vi "PH_Calorimeter_USB.get Data.vi"(0 "i ref in":refnum<vi>, 5 "error in (no error)":errorcluster) -> (14 "i ref out":refnum<vi>, 16 "raw data":dbl[][](array[numeric]), 17 "got Data":bool, 19 "error out":errorcluster)   [LabVIEW 2014, in "PH_Calorimeter_USB.lvlib"]
doc: "This VI interacts with the hardware. The data are taken and written to own attributes and the GUI."
uses:
  PH_Calorimeter_USB.lvlib
  <vilib>/DAQmx/create/channels.llb/DAQmx Create Channel (AI-Voltage-Basic).vi
  <vilib>/DAQmx/configure/timing.llb/DAQmx Timing (Sample Clock).vi
  <vilib>/DAQmx/read.llb/DAQmx Read (Analog 2D DBL NChan NSamp).vi
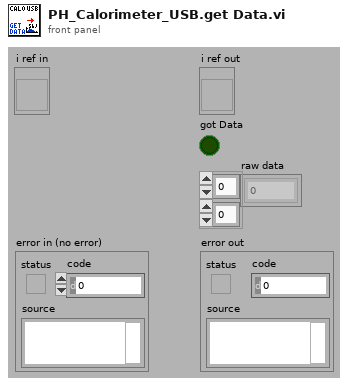
[diagram p1: front panel]
types:
  T1 = typedef "PH_Calorimeter_USB.lvlib/PH_Calorimeter_USB.i attribute.ctl" = cluster{"GUI Refs":cluster{"Delete":refnum<vi>, "Start":refnum<vi>, "Energy":refnum<vi>, "Calorimeter":refnum<vi>, "Trigger":refnum<vi>, "Calo Calibration":refnum<vi>, "Time Base":refnum<vi>, "Device":refnum<vi>, "Graph Raw Data":refnum<vi>, "Graph Result":refnum<vi>}, "DAQ Instance":string, "Data":dbl[][], "Controller Instance":string, "Energy [J]":dbl, "Calorimeter":T2, "Trigger":T3, "Time Base":T4, "Calo Calibration":T5, "Serial Number":string}
  T2 = typedef "PH_Calorimeter_USB.lvlib/PH_Calorimeter_USB.Calorimeter Settings.ctl" = cluster{"Channel":tag, "Min Value [V]":dbl, "Max Value  [V]":dbl}
  T3 = typedef "PH_Calorimeter_USB.lvlib/PH_Calorimeter_USB.Trigger Settings.ctl" = cluster{"Channel":tag, "Min Value [V]":dbl, "Max Value  [V]":dbl, "Level [V]":dbl, "Wait Time [s]":dbl, "Length [Samples]":i32}
  T4 = typedef "PH_Calorimeter_USB.lvlib/PH_Calorimeter_USB.Time Base Settings.ctl" = cluster{"Samples per Channel":i32, "Rate [Hz]":i32}
  T5 = typedef "PH_Calorimeter_USB.lvlib/PH_Calorimeter_USB.Calorimeter Calibration Settings.ctl" = cluster{"T 1/e [s]":dbl, "Sensitivity  [Vs/J]":dbl}
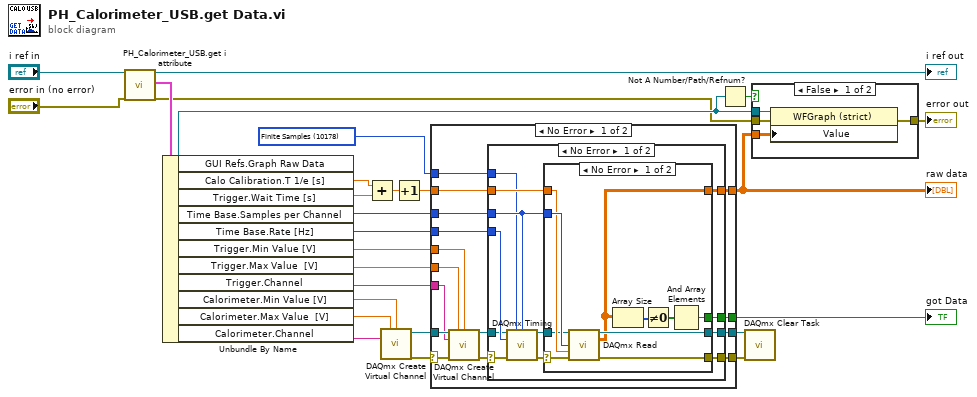
[diagram p0: block diagram]
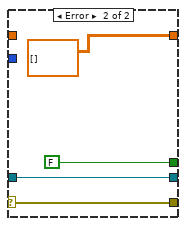
[diagram p2: hidden frame]
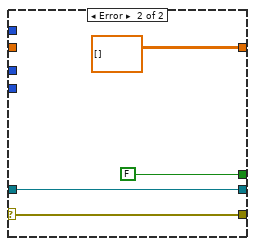
[diagram p3: hidden frame]
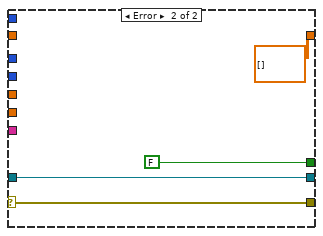
[diagram p4: hidden frame]
diagram:
  w3 = 10178 items=["Finite Samples"=10178, "Continuous Samples"=10123] ("sample mode")
  n1 = call "PH_Calorimeter_USB.get i attribute.vi"("i ref in"="i ref in", "error in (no error)"="error in (no error)") -> ("i ref out"=→"i ref out":refnum<vi>, "i attribute"=w16:T1, "error out"=w8:errorcluster)  [unwired: 15 in]
  n2 = Unbundle By Name(w16) -> ("GUI Refs.Graph Raw Data"=w27:refnum<vi>, "Calo Calibration.T 1/e [s]"=w25:dbl, "Trigger.Wait Time [s]"=w24:dbl, "Time Base.Samples per Channel"=w23:i32, "Time Base.Rate [Hz]"=w22:i32, "Trigger.Min Value [V]"=w21:dbl, "Trigger.Max Value  [V]"=w20:dbl, "Trigger.Channel"=w6:tag, "Calorimeter.Min Value [V]"=w19:dbl, "Calorimeter.Max Value  [V]"=w18:dbl, "Calorimeter.Channel"=w17:tag)
  n3 = Add(x=w25, y=w24) -> (x+y=w12:dbl)
  n4 = call-poly <vilib>:"DAQmx Create Virtual Channel.vi"("maximum value"=w18, "minimum value"=w19, "physical channels"=w17) -> ("task out"=w9:refnum<k21>, "error out"=w5:errorcluster)  [unwired: 11 in]
  n5 = Increment(x=w12) -> (x+1=w13:dbl)
  n6 = case shown="No Error" w5 {
    selector: w5 -> [w31 w76]
    tunnel: w23 -> [w42 _]
    tunnel: w22 -> [w41 _]
    tunnel: w21 -> [w40 _]
    tunnel: w20 -> [w39 _]
    tunnel: w13 -> [w38 _]
    tunnel: [w37 w75] -> w11
    tunnel: [w36 w76] -> w10
    tunnel: w9 -> [w35 w75]
    tunnel: [w34 dbl[][] [] ("data")] -> w7
    tunnel: w6 -> [w33 _]
    tunnel: [w29 FALSE] -> w4
    tunnel: w3 -> [w28 _]
    frame No Error {
      n7 = call-poly <vilib>:"DAQmx Create Virtual Channel.vi"("task in"=w35, "maximum value"=w39, "minimum value"=w40, "physical channels"=w33, "error in"=w31) -> ("task out"=w32:refnum<k21>, "error out"=w30:errorcluster)  [unwired: 9 in]
      n8 = case shown="No Error" w30 {
        selector: w30 -> [w46 w70]
        tunnel: w42 -> [w54 _]
        tunnel: w41 -> [w53 _]
        tunnel: w38 -> [w52 _]
        tunnel: [w51 w69] -> w37
        tunnel: [w50 w70] -> w36
        tunnel: [w49 dbl[][] [] ("data")] -> w34
        tunnel: w32 -> [w47 w69]
        tunnel: [w44 FALSE] -> w29
        tunnel: w28 -> [w43 _]
        frame No Error {
          n9 = call-poly <vilib>:"DAQmx Timing.vi"("task/channels in"=w47, "sample mode"=w43, "samples per channel"=w54, "rate"=w53, "error in"=w46) -> ("task out"=w48:refnum<k21>, "error out"=w45:errorcluster)  [unwired: 9 in]
          n10 = case shown="No Error" w45 {
            selector: w45 -> [w59 w68]
            tunnel: w54 -> [w64 _]
            tunnel: w52 -> [w63 _]
            tunnel: [w62 w67] -> w51
            tunnel: [w61 w68] -> w50
            tunnel: [w58 dbl[][] [] ("data")] -> w49
            tunnel: w48 -> [w60 w67]
            tunnel: [w55 FALSE] -> w44
            frame No Error {
              n11 = call-poly <vilib>:"DAQmx Read.vi"("task/channels in"=w60, "number of samples per channel"=w64, "timeout"=w63, "error in"=w59) -> ("task out"=w62:refnum<k21>, "data"=w58:dbl[][], "error out"=w61:errorcluster)  [unwired: 9 in]
              n12 = Array Size(array=w58) -> (size(s)=w57:i32[])
              n13 = Not Equal To 0?(x=w57) -> (x != 0?=w56:bool[])
              n14 = And Array Elements(Boolean array=w56) -> (logical AND=w55:bool)
            }
            frame Error {
            }
          }
        }
        frame Error {
        }
      }
    }
    frame Error {
    }
  }
  "got Data" <- w4
  "raw data" <- w7
  n15 = Not A Number/Path/Refnum?(number/path/refnum=w27) -> (NaN/Path/Refnum?=w26:bool)
  n16 = call <vilib>:"DAQmx Clear Task.vi"("task in"=w11, "error in"=w10) -> ()  [unwired: 13 in, 1 out]
  n17 = case shown="False" w26 {
    tunnel: w27 -> [w80 _]
    tunnel: w7 -> [w79 _]
    tunnel: w8 -> [w78 w81]
    tunnel: [w77 w81] -> w1
    frame False {
      n18 = property class="WFGraph (strict)"(reference=w80, error in=w78, "Value"=w79) -> (error out=w77:errorcluster)  [unwired: 1 out]
    }
    frame True {
    }
  }
  "error out" <- w1
